vi "Collect Boolean Array.vi"(6 "reset":bool, 7 "enable":bool=TRUE, 8 "error in":errorcluster, 10 "array size":u32=10, 11 "input":bool) -> (0 "error out":errorcluster, 1 "full":bool, 2 "points collected":i32=10, 3 "collected data":bool[](array[boolean]))   [LabVIEW 2012]
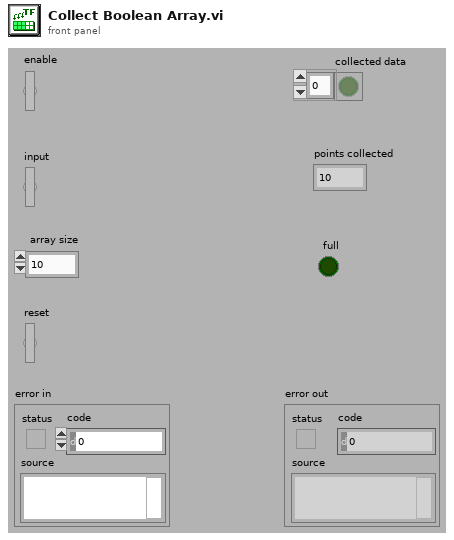
[diagram p1: front panel]
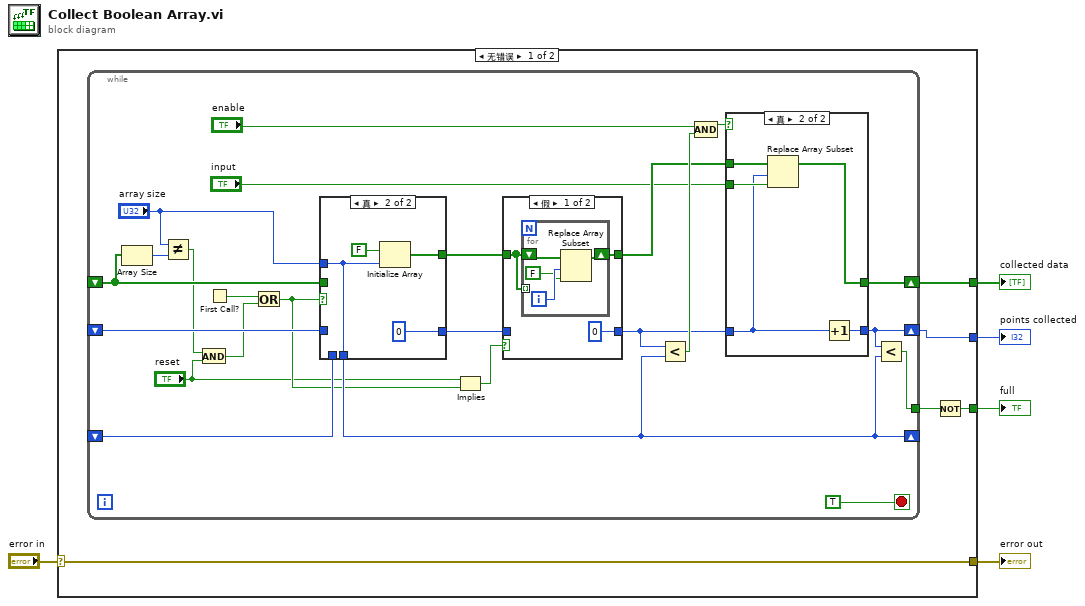
[diagram p0: block diagram]
diagram:
  n1 = case shown="无错误" "error in" {
    selector: "error in" -> [w6 w58]
    tunnel: [w10 _] -> w1
    tunnel: [w8 _] -> w2
    tunnel: [w7 _] -> w3
    tunnel: [w6 w58] -> w5
    frame No Error {
      n2 = while {
        shift-right: [w34] -> w10
        shift-left: _ -> [w18]
        shift-right: [w22] -> w7
        shift-left: _ -> [w32]
        shift-right: [w21] -> _
        shift-left: _ -> [w33]
        tunnel: [w20] -> w9
        stop <- TRUE stop-if-true
        n3 = Array Size(array=w18) -> (size(s)=w19:i32)
        n4 = Not Equal?(x="array size", y=w19) -> (x != y?=w16:bool)
        n5 = And(x=w16, y="reset") -> (x .and. y?=w15:bool)
        n6 = First Call?() -> (First Call?: T/F=w14:bool)
        n7 = Or(x=w14, y=w15) -> (x .or. y?=w13:bool)
        n8 = case shown="真" w13 {
          tunnel: "array size" -> [_ w54]
          tunnel: [w51 0] -> w28
          tunnel: [w52 w55] -> w26
          tunnel: [w53 w54] -> w21
          tunnel: w33 -> [w53 _]
          tunnel: w18 -> [w52 _]
          tunnel: w32 -> [w51 _]
          frame False {
          }
          frame True {
            n9 = Initialize Array(FALSE, w54) -> (w55:bool[])
          }
        }
        n10 = Implies(1:w13, 2:"reset") -> (0:w11:bool)
        n11 = case shown="假" w11 {
          tunnel: w28 -> [_ w43]
          tunnel: [0 w43] -> w27
          tunnel: w26 -> [w36 w42]
          tunnel: [w35 w42] -> w25
          frame False {
            n12 = for {
              tunnel: w36 -> [_] mode=indexing
              shift-right: [w39] -> w35
              shift-left: w36 -> [w38]
              i -> [w41]
              n13 = Replace Array Subset(array=w38, new element=FALSE, index=w41) -> (w39:bool[])
            }
          }
          frame True {
          }
        }
        n14 = Less?(x=w27, y=w21) -> (x < y?=w30:bool)
        n15 = Compound Arithmetic op=AND("enable", w30) -> (w31:bool)
        n16 = case shown="真" w31 {
          tunnel: "input" -> [_ w50]
          tunnel: w27 -> [w44 w47]
          tunnel: w25 -> [w45 w49]
          tunnel: [w45 w48] -> w34
          tunnel: [w44 w46] -> w22
          frame False {
          }
          frame True {
            n17 = Replace Array Subset(array=w49, new element=w50, index=w47) -> (w48:bool[])
            n18 = Increment(x=w47) -> (x+1=w46:i32)
          }
        }
        n19 = Less?(x=w22, y=w21) -> (x < y?=w20:bool)
      }
      n20 = Not(x=w9) -> (.not. x?=w8:bool)
    }
    frame Error {
    }
  }
  "collected data" <- w1
  "full" <- w2
  "points collected" <- w3
  "error out" <- w5
